vi "IBM4_Read_all_Bytes.vi"(4 "error in (no error)":errorcluster, 6 "milliseconds to wait":u32=10, 7 "VISA Refnum in":refnum<visa-resource-name>="COM12") -> (0 "error out":errorcluster, 2 "String":string="BRead0:1\r\nOutput 0 = 416 \r\n", 3 "VISA Refnum out":refnum<visa-resource-name>="COM12")   [LabVIEW 2021, in "IBM4.lvlib"]
uses:
  <instrlib>/IBM4/IBM4.lvlib
panel:
  out "Iteration":i32
  out "Array":u32[](array[numeric])
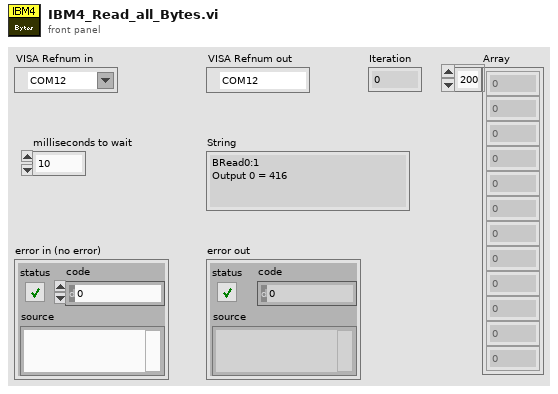
[diagram p1: front panel]
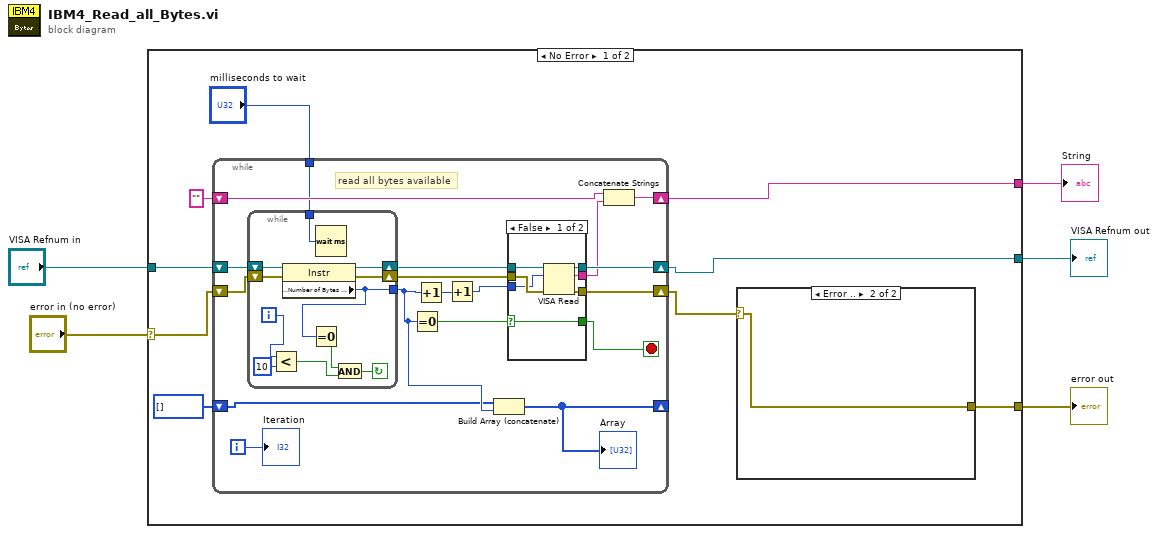
[diagram p0: block diagram]
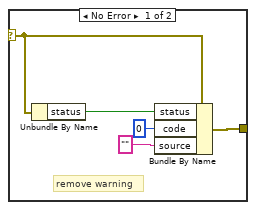
[diagram p2: hidden frame]
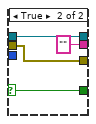
[diagram p3: hidden frame]
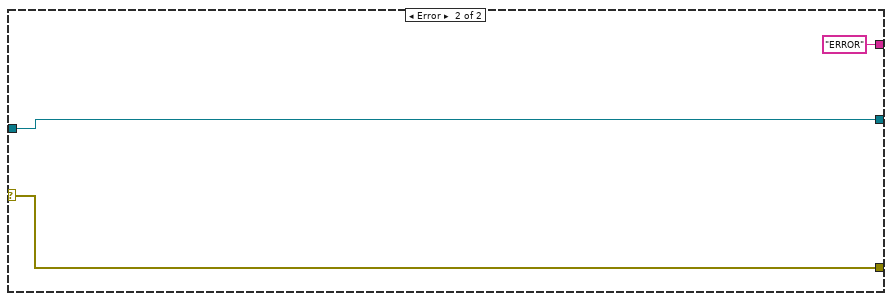
[diagram p4: hidden frame]
diagram:
  n1 = case shown="No Error" "error in (no error)" {
    selector: "error in (no error)" -> [w7 w62]
    tunnel: [w13 "ERROR"] -> w5
    tunnel: [w12 w63] -> w4
    tunnel: "VISA Refnum in" -> [w11 w63]
    tunnel: [w9 w62] -> w2
    frame No Error {
      n2 = while {
        shift-right: [w38] -> w12
        shift-left: w11 -> [w36]
        shift-right: [w37] -> w10
        shift-left: w7 -> [w34]
        shift-right: [w32] -> w13
        shift-left: "" -> [w30]
        tunnel: "milliseconds to wait" -> [w25]
        shift-right: [w22] -> _
        shift-left: u32[] [] -> [w23]
        i -> [w21]
        stop <- w28 stop-if-true
        # "read all bytes available"
        n3 = while {
          tunnel: [w56] -> w24
          shift-right: [w59] -> w35
          shift-left: w36 -> [w60]
          shift-right: [w57] -> w33
          shift-left: w34 -> [w58]
          tunnel: w25 -> [w51]
          i -> [w50]
          stop <- w54 continue-if-true
          n4 = Less?(x=w50, y=10) -> (x < y?=w53:bool)
          n5 = property class="Instr"(reference=w60, error in=w58) -> (reference out=w59:refnum<visa-resource-name>, error out=w57:errorcluster, "Serial Settings:Number of Bytes at Serial Port"=w56:u32)
          n6 = Equal To 0?(x=w56) -> (x = 0?=w52:bool)
          n7 = Wait (ms)(milliseconds to wait=w51) -> ()  [unwired: 1 out]
          n8 = And(x=w52, y=w53) -> (x .and. y?=w54:bool)
        }
        n9 = Equal To 0?(x=w24) -> (x = 0?=w29:bool)
        n10 = Increment(x=w24) -> (x+1=w27:u32)
        n11 = Increment(x=w27) -> (x+1=w26:u32)
        n12 = Build Array (concatenate)(w23, w24) -> (w22:u32[])
        "Array" <- w22
        n13 = case shown="False" w29 {
          selector: w29 -> [w39 w48]
          tunnel: [w45 w49] -> w38
          tunnel: [w44 w47] -> w37
          tunnel: w35 -> [w43 w49]
          tunnel: w33 -> [w42 w47]
          tunnel: [w41 "" ("read buffer")] -> w31
          tunnel: w26 -> [w40 _]
          tunnel: [w39 w48] -> w28
          frame False {
            n14 = VISA Read(VISA resource name=w43, byte count=w40, error in (no error)=w42) -> (VISA resource name out=w45:refnum<visa-resource-name>, read buffer=w41:string, error out=w44:errorcluster)  [unwired: 1 out]
          }
          frame True {
          }
        }
        n15 = Concatenate Strings(w30, w31) -> (w32:string)
        "Iteration" <- w21
      }
      n16 = case shown="Error .." w10 {
        selector: w10 -> [w19 w20]
        tunnel: [w15 w20] -> w9
        frame No Error {
          # "remove warning"
          n17 = Unbundle By Name(w19) -> ("status"=w18:bool)
          n18 = Bundle By Name(cluster=w19, "status"=w18, "code"=0, "source"="") -> (w15:errorcluster)
        }
        frame Error {
        }
      }
    }
    frame Error {
    }
  }
  "String" <- w5
  "VISA Refnum out" <- w4
  "error out" <- w2
